vi "Byte61_68 (SubVI).vi"(3 "Input String":string) -> (0 "Voltage Alert":T1, 1 "Cluster":T2={"Input (TRU) voltage value "=0.0, "TRU Temperature value "=0.0, "EPS Mode"=enum."Maintenance Mode"}, 2 "Enum":T3(ring)=enum."Operational Mode")   [LabVIEW 2024]
panel:
  # "SAMPLE: \nAAAA AAAA AAAA AAAA AAAA AAAA AAAA AAAA AAAA AAAA AAAA AAAA AAAA AAAA AAAA AAAA AAAA AAAA AAAA AAAA AAAA AAAA AAAA AAAA AAAA AAAA AAAA AAAA AAAA AAAA AA2F 1111 AAAA C900 33"
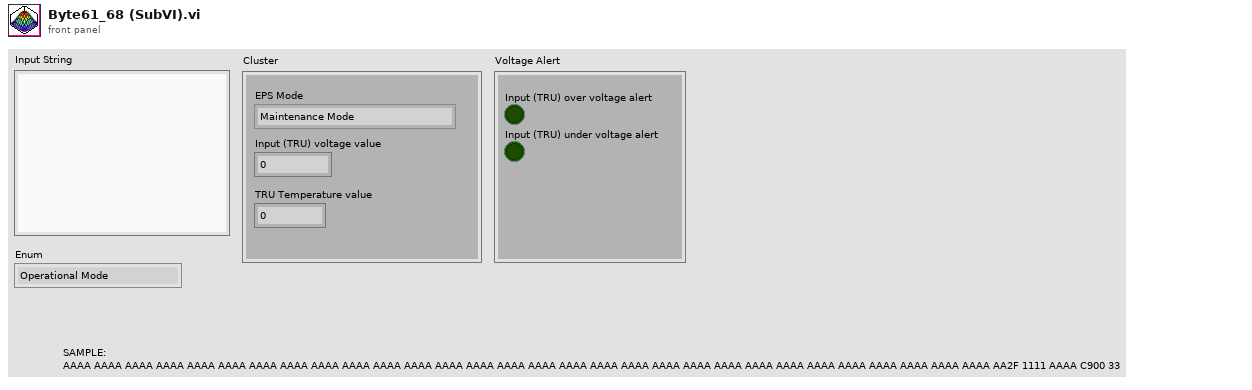
[diagram p1: front panel]
types:
  T1 = cluster{"Input (TRU) over voltage alert":bool, "Input (TRU) under voltage alert":bool}
  T2 = cluster{"Input (TRU) voltage value ":dbl, "TRU Temperature value ":dbl, "EPS Mode":enum16{"Power-On Mode", "Maintenance Mode", "Operational Mode", "Emergency Mode"}}
  T3 = enum8{"Power-On Mode", "Maintenance Mode", "Operational Mode", "Emergency Mode"}
  T4 = enum16{"Power-On Mode", "Maintenance Mode", "Operational Mode", "Emergency Mode"}
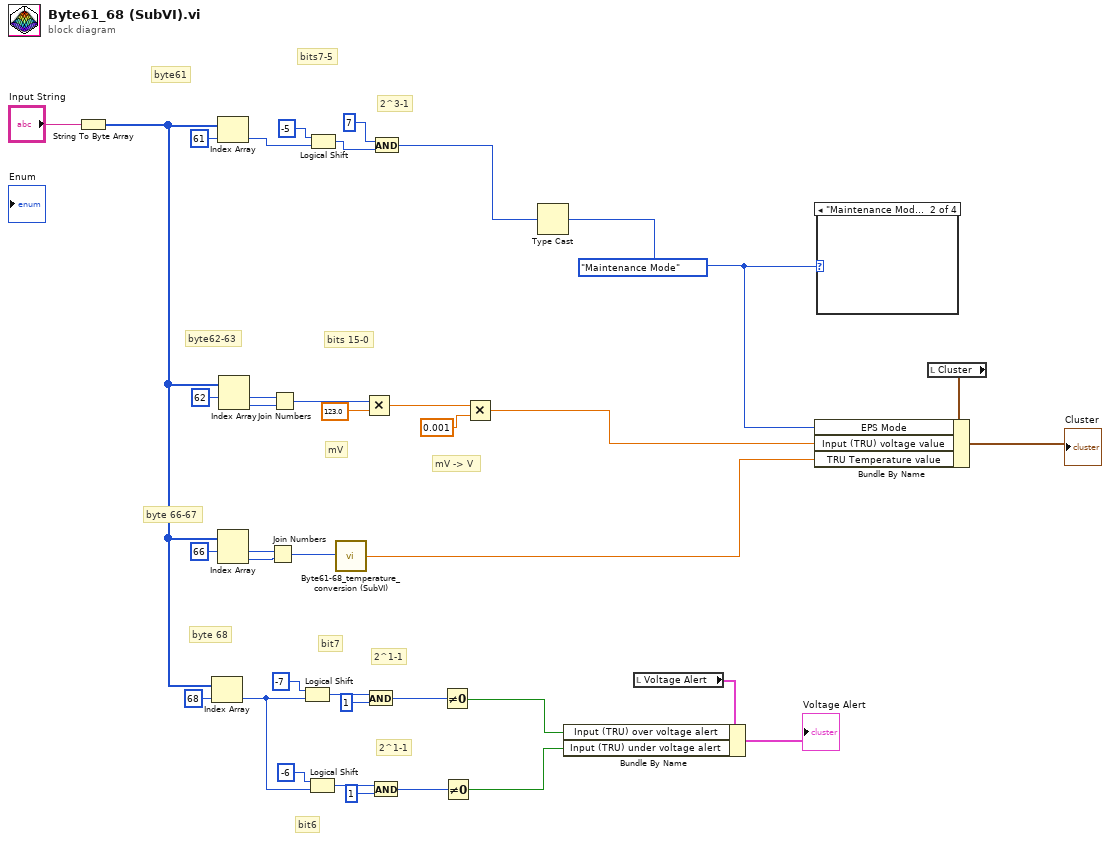
[diagram p0: block diagram]
diagram:
  w5 = T4."Maintenance Mode"
  # "2^1-1"
  # "bit6"
  # "byte 68"
  # "2^1-1"
  # "bit7"
  # "byte 66-67"
  # "mV -> V"
  # "mV"
  # "bits 15-0"
  # "byte62-63"
  # "2^3-1"
  # "bits7-5"
  # "byte61"
  n1 = String To Byte Array(string="Input String") -> (unsigned byte array=w20:u8[])
  n2 = Index Array "Index Array"(array=w20, index=68) -> (element=w16:u8)
  n3 = Index Array "Index Array"(array=w20, index=61) -> (element=w36:u8)
  n4 = Index Array "Index Array"(array=w20, index #1=66 ("index")) -> (element #1=w25:u8, element #2=w26:u8)  [unwired: 1 in]
  n5 = Index Array "Index Array"(array=w20, index #1=62 ("index")) -> (element #1=w33:u8, element #2=w32:u8)  [unwired: 1 in]
  n6 = Join Numbers(hi=w25, lo=w26) -> ((hi.lo)=w11:u16)
  n7 = Join Numbers(hi=w33, lo=w32) -> ((hi.lo)=w28:u16)
  n8 = Logical Shift(y=i16 -7, x=w16) -> (x << y=w22:u8)
  n9 = Logical Shift(y=i16 -6, x=w16) -> (x << y=w18:u8)
  n10 = Logical Shift(y=i16 -5, x=w36) -> (x << y=w9:u8)
  n11 = call "Byte61-68_temperature_conversion (SubVI).vi"("Numeric"=w11) -> ("Control Card Temperature value"=w3:dbl)
  n12 = Multiply(x=w28, y=123.0) -> (x*y=w30:dbl)
  n13 = And(x=w22, y=u8 1) -> (x .and. y?=w15:u8)
  n14 = And(x=w18, y=u8 1) -> (x .and. y?=w14:u8)
  n15 = And(x=u8 7, y=w9) -> (x .and. y?=w10:u8)
  n16 = Not Equal To 0?(x=w15) -> (x != 0?=w13:bool)
  n17 = Not Equal To 0?(x=w14) -> (x != 0?=w12:bool)
  n18 = Multiply(x=w30, y=0.001) -> (x*y=w4:dbl)
  n19 = Type Cast(type=w5, x=w10) -> ()  [unwired: 1 out]
  n20 = local read "Voltage Alert"() -> (w2:T1)
  n21 = Bundle By Name(cluster=w2, "Input (TRU) over voltage alert"=w13, "Input (TRU) under voltage alert"=w12) -> (→"Voltage Alert":T1)
  n22 = case shown="\"Maintenance Mode\"" w5 {
    frame "Power-On Mode", Default {
    }
    frame "Maintenance Mode" {
    }
    frame "Operational Mode" {
    }
    frame "Emergency Mode" {
    }
  }
  n23 = local read "Cluster"() -> (w7:T2)
  n24 = Bundle By Name(cluster=w7, "EPS Mode"=w5, "Input (TRU) voltage value"=w4, "TRU Temperature value"=w3) -> (→"Cluster":T2)
